vi "To_CP_testing.vi"(0 "Enum":enum16{""}(ring), 5 "FGFG":bool, 6 "DUPA":dbl) -> ()   [LabVIEW 2015]
doc: "Test"
panel:
  in  "fdgf":string
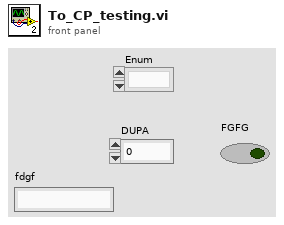
[diagram p1: front panel]
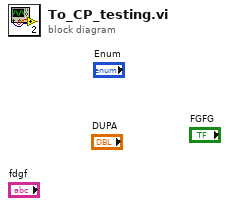
[diagram p0: block diagram]
diagram:
